vi "Get all Dependencies.vi"(0 "Measurement paths":path[](array[path]), 11 "error in (no error)":errorcluster) -> (4 "All dependencies":path[][](array[path]), 6 "Instrument containing subVIs":path[][](array[path]), 15 "error out":errorcluster)   [LabVIEW 2021, in "Multiple Converter.lvlib"]
uses:
  Multiple Converter.lvlib
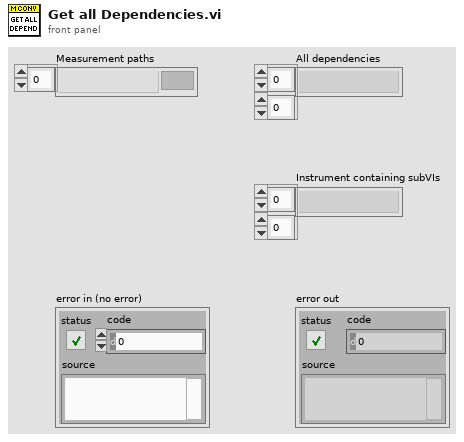
[diagram p1: front panel]
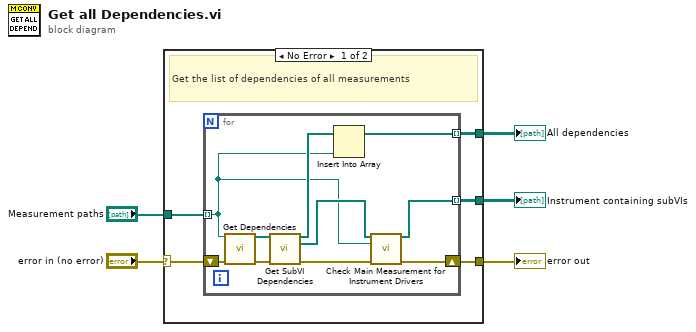
[diagram p0: block diagram]
diagram:
  n1 = case shown="No Error" "error in (no error)" {
    selector: "error in (no error)" -> [w7 w21]
    tunnel: "Measurement paths" -> [w10 _]
    tunnel: [w9 _] -> w4
    tunnel: [w8 w21] -> w3
    tunnel: [w6 _] -> w2
    frame No Error {
      # "Get the list of dependencies of all measurements"
      n2 = for {
        shift-right: [w13] -> w8
        shift-left: w7 -> [w20]
        tunnel: w10 -> [w14] mode=indexing
        tunnel: [w16] -> w9 mode=indexing
        tunnel: [w11] -> w6 mode=indexing
        n3 = call "Get Dependencies.vi"("VI path"=w14, "error in (no error)"=w20) -> ("Existing dependencies"=w18:path[], "error out"=w19:errorcluster)  [unwired: 12 in]
        n4 = call "Get SubVI Dependencies.vi"("Dependency Paths"=w18, "error in (no error)"=w19) -> ("All dependencies"=w17:path[], "Instrument containing subVIs"=w15:path[], "error out"=w12:errorcluster)  [unwired: 11 in]
        n5 = Insert Into Array(array=w17, new element=w14) -> (w16:path[])  [unwired: 1 in]
        n6 = call "Check Main Measurement for Instrument Drivers.vi"("Instrument containing subVIs"=w15, "Measurement path"=w14, "error in (no error)"=w12) -> ("Instrument containing subVIs Out"=w11:path[], "error out"=w13:errorcluster)  [unwired: 11 in]
      }
    }
    frame Error {
      # "Pass"
    }
  }
  "All dependencies" <- w4
  "error out" <- w3
  "Instrument containing subVIs" <- w2
